vi "Configure Power.vi"(0 "VISA resource name":refnum<visa-resource-name>, 1 "Power Reference (0 dBm)":dbl, 2 "Enable Power Reference (F:Disable)":bool, 5 "Power (-130 dBm)":dbl=-130.0, 7 "Power Offset (0 dB)":dbl, 9 "Attenuator Auto Mode (T:Enable)":bool=TRUE, 11 "error in (no error)":errorcluster, 12 "Enable Attenuator Bypass (F:Disable)":bool, 13 "Attenuation Level (115 dB)":dbl=115.0) -> (4 "VISA resource name out":refnum<visa-resource-name>, 15 "error out":errorcluster)   [LabVIEW 2011, in "Agilent PSG MXG Series.lvlib"]
doc: "Configures RF output power."
uses:
  Agilent PSG MXG Series.lvlib
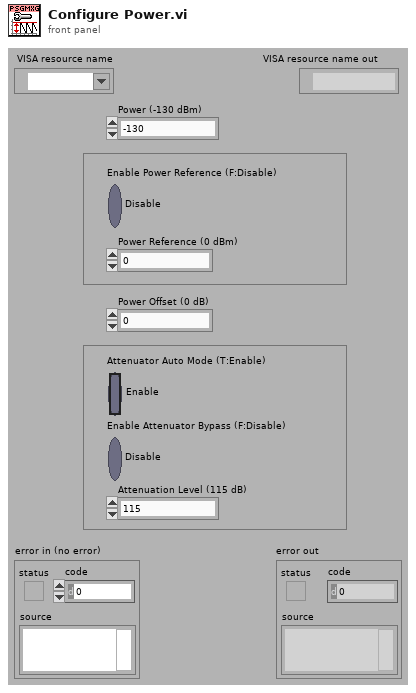
[diagram p1: front panel]
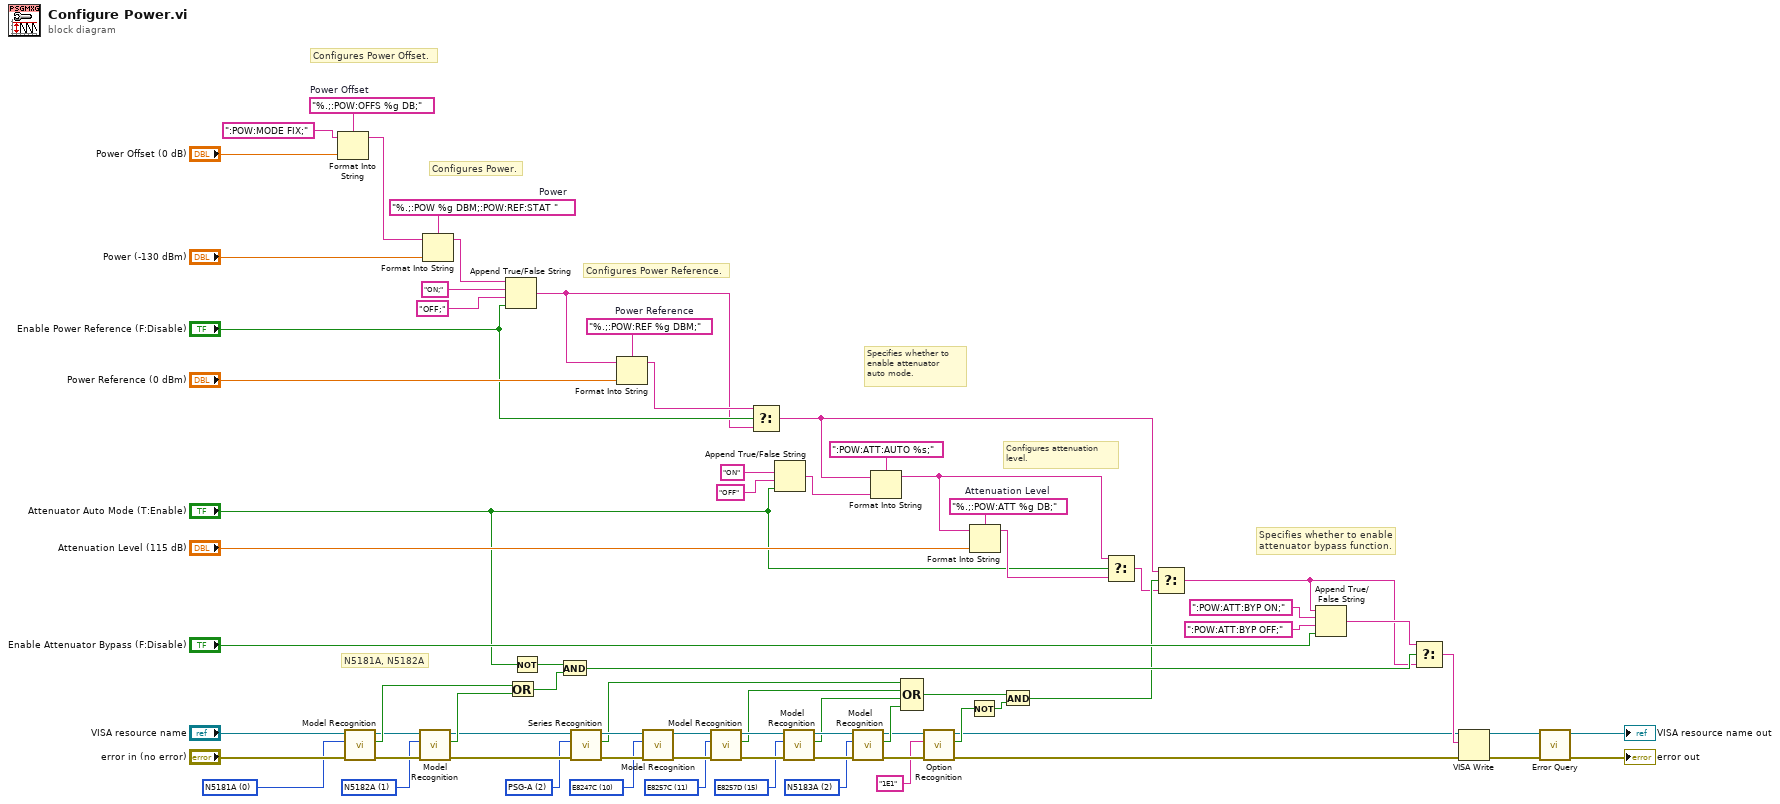
[diagram p0: block diagram]
diagram:
  w22 = u16 2 items=["N5181A"=0, "N5182A"=1, "N5183A"=2, "E8241A"=5, "E8244A"=6, "E8251A"=7, "E8254A"=8, "E8247C"=10, "E8257C"=11, "E8267C"=12, "E8257D"=15, "E8267D"=16] ("Model Type (0: N5181A)")
  w25 = u16 15 items=["N5181A"=0, "N5182A"=1, "N5183A"=2, "E8241A"=5, "E8244A"=6, "E8251A"=7, "E8254A"=8, "E8247C"=10, "E8257C"=11, "E8267C"=12, "E8257D"=15, "E8267D"=16] ("Model Type (0: N5181A)")
  w28 = u16 11 items=["N5181A"=0, "N5182A"=1, "N5183A"=2, "E8241A"=5, "E8244A"=6, "E8251A"=7, "E8254A"=8, "E8247C"=10, "E8257C"=11, "E8267C"=12, "E8257D"=15, "E8267D"=16] ("Model Type (0: N5181A)")
  w31 = u16 10 items=["N5181A"=0, "N5182A"=1, "N5183A"=2, "E8241A"=5, "E8244A"=6, "E8251A"=7, "E8254A"=8, "E8247C"=10, "E8257C"=11, "E8267C"=12, "E8257D"=15, "E8267D"=16] ("Model Type (0: N5181A)")
  w34 = u16 2 items=["MXG", "PSG", "PSG-A", "PSG-C", "PSG-D"] ("Series Type (0: MXG)")
  w38 = u16 1 items=["N5181A"=0, "N5182A"=1, "N5183A"=2, "E8241A"=5, "E8244A"=6, "E8251A"=7, "E8254A"=8, "E8247C"=10, "E8257C"=11, "E8267C"=12, "E8257D"=15, "E8267D"=16] ("Model Type (0: N5181A)")
  w43 = u16 0 items=["N5181A"=0, "N5182A"=1, "N5183A"=2, "E8241A"=5, "E8244A"=6, "E8251A"=7, "E8254A"=8, "E8247C"=10, "E8257C"=11, "E8267C"=12, "E8257D"=15, "E8267D"=16] ("Model Type (0: N5181A)")
  w52 = "%.;:POW:OFFS %g DB;"  # Power Offset
  w66 = "%.;:POW:ATT %g DB;"  # Attenuation Level
  w69 = "%.;:POW:REF %g DBM;"  # Power Reference
  w74 = "%.;:POW %g DBM;:POW:REF:STAT "  # Power
  # "N5181A, N5182A"
  # "Specifies whether to enable\nattenuator bypass function."
  # "Configures attenuation\nlevel."
  # "Specifies whether to\nenable attenuator\nauto mode."
  # "Configures Power Offset."
  # "Configures Power Reference."
  # "Configures Power."
  n1 = Format Into String(format string=w52, initial string=":POW:MODE FIX;" ("Power Mode"), "Power Offset (0 dB)") -> (resulting string=w1:string)  [unwired: 1 in, 1 out]
  n2 = call "Model Recognition.vi"("error in (no error)"="error in (no error)", "Model Type (0: N5181A)"=w43, "VISA resource name"="VISA resource name") -> ("error out"=w39:errorcluster, "Is Model Correct"=w41:bool, "VISA resource name out"=w40:refnum<visa-resource-name>)  [unwired: 6 in]
  n3 = call "Model Recognition.vi"("error in (no error)"=w39, "Model Type (0: N5181A)"=w38, "VISA resource name"=w40) -> ("error out"=w35:errorcluster, "Is Model Correct"=w37:bool, "VISA resource name out"=w36:refnum<visa-resource-name>)  [unwired: 6 in]
  n4 = Format Into String(format string=w74, initial string=w1, "Power (-130 dBm)") -> (resulting string=w72:string)  [unwired: 1 in, 1 out]
  n5 = Append True/False String(1:"Enable Power Reference (F:Disable)", 2:"OFF;" ("false string"), 3:"ON;" ("true string"), 4:w72) -> (0:w54:string)
  n6 = Or(x=w41, y=w37) -> (x .or. y?=w42:bool)
  n7 = Not(x="Attenuator Auto Mode (T:Enable)") -> (.not. x?=w50:bool)
  n8 = And(x=w50, y=w42) -> (x .and. y?=w57:bool)
  n9 = call "Series Recognition.vi"("error in (no error)"=w35, "Series Type (0: MXG)"=w34, "VISA resource name"=w36) -> ("error out"=w32:errorcluster, "Is Series Correct"=w21:bool, "VISA resource name out"=w33:refnum<visa-resource-name>)  [unwired: 6 in]
  n10 = Format Into String(format string=w69, initial string=w54, "Power Reference (0 dBm)") -> (resulting string=w55:string)  [unwired: 1 in, 1 out]
  n11 = call "Model Recognition.vi"("error in (no error)"=w32, "Model Type (0: N5181A)"=w31, "VISA resource name"=w33) -> ("error out"=w29:errorcluster, "VISA resource name out"=w30:refnum<visa-resource-name>)  [unwired: 6 in, 1 out]
  n12 = call "Model Recognition.vi"("error in (no error)"=w29, "Model Type (0: N5181A)"=w28, "VISA resource name"=w30) -> ("error out"=w26:errorcluster, "Is Model Correct"=w20:bool, "VISA resource name out"=w27:refnum<visa-resource-name>)  [unwired: 6 in]
  n13 = Select(t=w55, s="Enable Power Reference (F:Disable)", f=w54) -> (s? t:f=w3:string)
  n14 = Append True/False String(1:"Attenuator Auto Mode (T:Enable)", 2:"OFF" ("false string"), 3:"ON" ("true string")) -> (0:w12:string)  [unwired: 1 in]
  n15 = call "Model Recognition.vi"("error in (no error)"=w26, "Model Type (0: N5181A)"=w25, "VISA resource name"=w27) -> ("error out"=w23:errorcluster, "Is Model Correct"=w19:bool, "VISA resource name out"=w24:refnum<visa-resource-name>)  [unwired: 6 in]
  n16 = call "Model Recognition.vi"("error in (no error)"=w23, "Model Type (0: N5181A)"=w22, "VISA resource name"=w24) -> ("error out"=w16:errorcluster, "Is Model Correct"=w18:bool, "VISA resource name out"=w17:refnum<visa-resource-name>)  [unwired: 6 in]
  n17 = Format Into String(format string=":POW:ATT:AUTO %s;", initial string=w3, w12) -> (resulting string=w11:string)  [unwired: 1 in, 1 out]
  n18 = Compound Arithmetic op=OR(w21, w20, w19, w18) -> (w14:bool)
  n19 = call "Option Recognition.vi"("error in (no error)"=w16, "Option (\"\")"="1E1" ("Option (\"\")"), "VISA resource name"=w17) -> ("error out"=w4:errorcluster, "Is Option Installed"=w8:bool, "VISA resource name out"=w5:refnum<visa-resource-name>)  [unwired: 6 in]
  n20 = Not(x=w8) -> (.not. x?=w9:bool)
  n21 = Format Into String(format string=w66, initial string=w11, "Attenuation Level (115 dB)") -> (resulting string=w64:string)  [unwired: 1 in, 1 out]
  n22 = And(x=w14, y=w9) -> (x .and. y?=w10:bool)
  n23 = Select(t=w11, s="Attenuator Auto Mode (T:Enable)", f=w64) -> (s? t:f=w7:string)
  n24 = Select(t=w3, s=w10, f=w7) -> (s? t:f=w6:string)
  n25 = Append True/False String(1:"Enable Attenuator Bypass (F:Disable)", 2:":POW:ATT:BYP OFF;" ("true string"), 3:":POW:ATT:BYP ON;" ("true string"), 4:w6) -> (0:w48:string)
  n26 = Select(t=w48, s=w57, f=w6) -> (s? t:f=w59:string)
  n27 = VISA Write(VISA resource name=w5, write buffer=w59, error in (no error)=w4) -> (VISA resource name out=w61:refnum<visa-resource-name>, error out=w60:errorcluster)  [unwired: 1 out]
  n28 = call "Error Query.vi"("error in (no error)"=w60, "VISA resource name"=w61) -> ("error out"=→"error out":errorcluster, "VISA resource name out"=→"VISA resource name out":refnum<visa-resource-name>)  [unwired: 6 in, 2 out]
